vi "Get_Channel_averages.vi"(0 "Desired Ch Names":string[](array[string]), 1 "Averaging time (mins)":dbl=5.0 format="%.2f", 2 "End Offset Sec (0)":dbl format="%.2f") -> (3 "Comments":string[](array[string]), 4 "Values":string[](array[string]), 5 "number":dbl[](array[numeric]) format="%.3f")   [LabVIEW 2010]
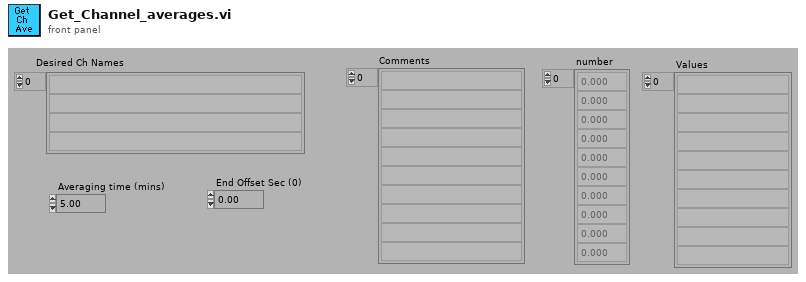
[diagram p1: front panel]
types:
  T1 = typedef "Ch_description_ADAM.ctl" = cluster{"Ch Name":string, "Type":T2, "Function":T3, "Ch State":T4, "Calibration type":T5, "A":dbl, "B":dbl, "C":dbl, "D":dbl, "Comments":string, "Address":T6, "String":string, "Duty":u16}
  T2 = typedef "Module_type_ADAM.ctl" = enum16{"4011", "4012", "4013", "4014", "4016", "4017", "4018", "4021", "4050", "4052", "4053", "4060", "4080", "5000", "5017", "5018", "5024", "5051", "5056", "5060", "6060", "Tracker", "WEST", "GILL", "JEM", "VICI", "Vaisala", "DRUCK", "Run VI Named:", "IR2100", "PPT", "Comparator", "VIRTUAL", "Hold Value", "Read A", "Read Ch", "Coded", "Client Info", "Web Client", "X10", "Test"}
  T3 = typedef "Function_ADAM.ctl" = enum16{"Analogue Input", "Digital Input", "Event counter", "Event rate", "Analogue Output", "Digital Output", "Relay Output"}
  T4 = typedef "Channel_State.ctl" = enum16{"On", "Off", "Always On", "Always Off"}
  T5 = typedef "Calib_type_ADAM.ctl" = enum16{"Raw", "Bx + A", "Cx^2 + Bx + A", "Dx^3 + Cx^2 + Bx + A", "In Band", "Hi-Tec Q", "Hi-Tec M_dot", "Text"}
  T6 = typedef "Address.ctl" = cluster{"Main":i32, "Ch.":i32, "Sub":i32, "Port Name":string}
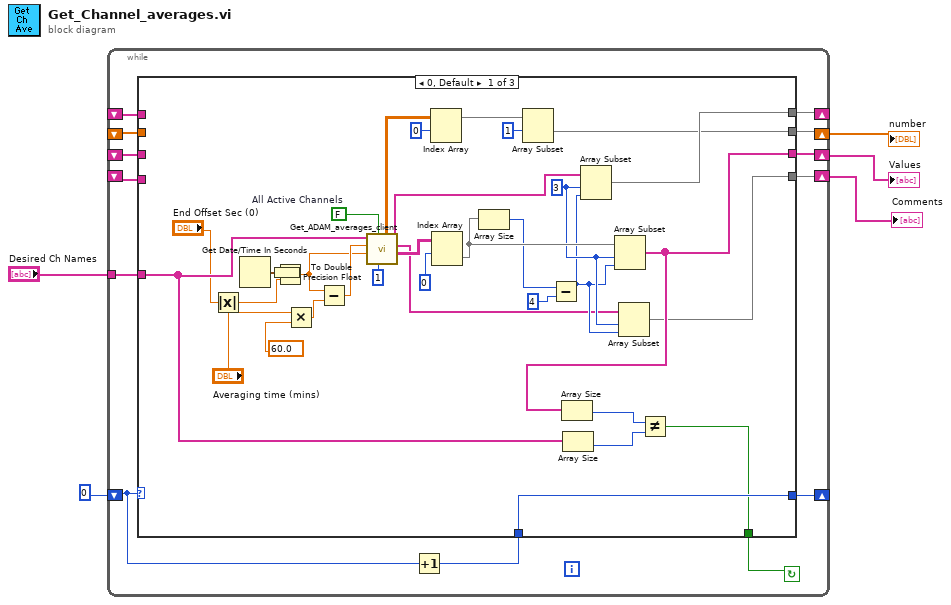
[diagram p0: block diagram]
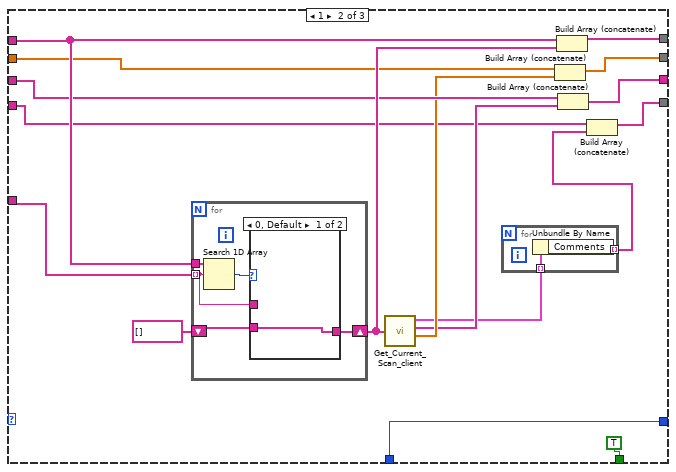
[diagram p2: hidden frame]
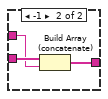
[diagram p3: hidden frame]
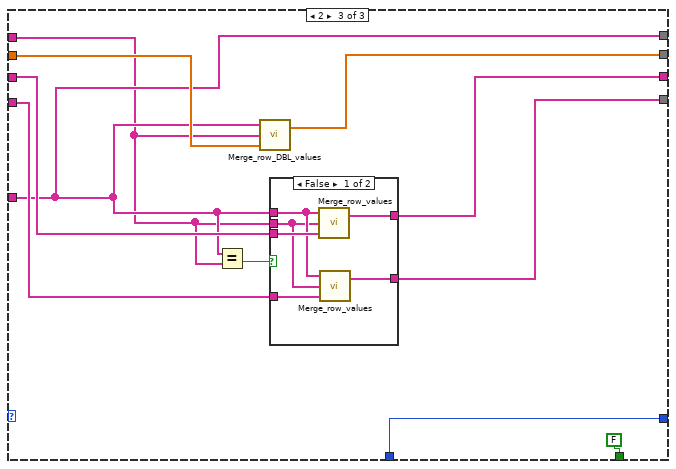
[diagram p4: hidden frame]
diagram:
  n1 = while {
    shift-left: _ -> [w6]
    shift-right: [w7] -> w1
    shift-left: 0 -> [w13]
    shift-right: [w14] -> _
    shift-left: _ -> [w8]
    shift-right: [w15] -> w2
    shift-left: _ -> [w9]
    shift-right: [w16] -> w3
    shift-left: _ -> [w10]
    shift-right: [w17] -> _
    tunnel: "Desired Ch Names" -> [w18]
    stop <- w11 continue-if-true
    n2 = Increment(x=w13) -> (x+1=w12:i32)
    n3 = case shown="0, Default" w13 {
      tunnel: w18 -> [w33 w68 w82]
      tunnel: [w32 w58 w88] -> w15
      tunnel: [w38 w64 w82] -> w17
      tunnel: [w34 w59 w89] -> w16
      tunnel: [w29 w56 w87] -> w14
      tunnel: w12 -> [w29 w56 w87]
      tunnel: [w28 TRUE FALSE] -> w11
      tunnel: w10 -> [_ w66 w81]
      tunnel: w9 -> [_ w63 w90]
      tunnel: w8 -> [_ w62 w85]
      tunnel: [w24 w52 w83] -> w7
      tunnel: w6 -> [_ w54 w84]
      frame 0, Default {
        w37 = FALSE  # All Active Channels
        w27 = 3 ("Array Index")
        n4 = Absolute Value(x="End Offset Sec (0)") -> (abs(x)=w20:dbl)
        n5 = Get Date/Time In Seconds() -> (seconds since 1Jan1904=w19:timestamp)
        n6 = To Double Precision Float(number=w19) -> (double precision float=w23:dbl)
        n7 = Subtract(x=w23, y=w20) -> (x-y=w21:dbl)
        n8 = Multiply(x="Averaging time (mins)", y=60.0) -> (x*y=w47:dbl)
        n9 = Subtract(x=w21, y=w47) -> (x-y=w50:dbl)
        n10 = call "Get_ADAM_averages_client.vi"("No of averages"=1, "All Active Channels"=w37, "End time"=w21, "Start time"=w50, "ADAM Ch Names"=w33) -> ("Values"=w42:string[][], "Comments"=w25:string[], "Titles"=w39:string[], "DBL values"=w40:dbl[][])  [unwired: 3 out]
        n11 = Index Array(array=w40, index (row)=0) -> (element=w36:dbl[])  [unwired: 1 in]
        n12 = Index Array(array=w42, index (row)=0) -> (element=w45:string[])  [unwired: 1 in]
        n13 = Array Size(array=w45) -> (size(s)=w44:i32)
        n14 = Array Subset(array=w36, index=1 ("Array Index")) -> (w34:dbl[])  [unwired: 1 in]
        n15 = Subtract(x=w44, y=4) -> (x-y=w26:i32)
        n16 = Array Size(array=w33) -> (size(s)=w31:i32)
        n17 = Array Subset(array=w39, index=w27, length=w26) -> (w38:string[])
        n18 = Array Subset(array=w45, index=w27, length=w26) -> (w32:string[])
        n19 = Array Size(array=w32) -> (size(s)=w30:i32)
        n20 = Array Subset(array=w25, index=w27, length=w26) -> (w24:string[])
        n21 = Not Equal?(x=w30, y=w31) -> (x != y?=w28:bool)
      }
      frame 1 {
        n22 = for {
          tunnel: w66 -> [w75]
          tunnel: w68 -> [w71] mode=indexing
          shift-right: [w72] -> w65
          shift-left: string[] [] -> [w73]
          n23 = Search 1D Array(1D array=w75, element=w71) -> (index of element=w74:i32)  [unwired: 1 out]
          n24 = case shown="0, Default" w74 {
            tunnel: w73 -> [w76 w79]
            tunnel: [w76 w78] -> w72
            tunnel: w71 -> [_ w77]
            frame 0, Default {
            }
            frame -1 {
              n25 = Build Array (concatenate)(w79, w77) -> (w78:string[])
            }
          }
        }
        n26 = call "Get_Current_Scan_client.vi"("ADAM Ch Names"=w65) -> ("Ch Description Array"=w55:T1[], "String values"=w60:string[], "Numerical Values"=w61:dbl[])  [unwired: 1 out]
        n27 = for {
          tunnel: w55 -> [w70] mode=indexing
          tunnel: [w69] -> w53 mode=indexing
          n28 = Unbundle By Name(w70) -> ("Comments"=w69:string)
        }
        n29 = Build Array (concatenate)(w63, w61) -> (w59:dbl[])
        n30 = Build Array (concatenate)(w66, w65) -> (w64:string[])
        n31 = Build Array (concatenate)(w62, w60) -> (w58:string[])
        n32 = Build Array (concatenate)(w54, w53) -> (w52:string[])
      }
      frame 2 {
        n33 = Equal?(x=w82, y=w81) -> (x = y?=w80:bool)
        n34 = call "Merge_row_DBL_values.vi"("Present Row values"=w90, "Present Channels"=w81, "Desired Channels"=w82) -> ("Desired Row values"=w89:dbl[])  [unwired: 1 out]
        n35 = case shown="False" w80 {
          tunnel: [w96 w98] -> w88
          tunnel: w85 -> [w95 w98]
          tunnel: w84 -> [w94 w97]
          tunnel: [w93 w97] -> w83
          tunnel: w82 -> [w92 _]
          tunnel: w81 -> [w91 _]
          frame False {
            n36 = call "Merge_row_values.vi"("Present Row values"=w95, "Present Channels"=w91, "Desired Channels"=w92) -> ("Desired Row values"=w96:string[])  [unwired: 1 out]
            n37 = call "Merge_row_values.vi"("Present Row values"=w94, "Present Channels"=w91, "Desired Channels"=w92) -> ("Desired Row values"=w93:string[])  [unwired: 1 out]
          }
          frame True {
          }
        }
      }
    }
  }
  "number" <- w3
  "Values" <- w2
  "Comments" <- w1
